vi "Basic ITC-Init2.vi"(0 "Connection Details":T6={"VISA resource name"="", "Comms Layer"=enum."Ethernet TCP/IP", "IP Address"="", "Serial Configuration"={"Baud Rate"=115200, "Parity"=0, "Data Bits"=8, "Stop Bits"=10, "Flow Control"=0}, "ISOBUS address"=-1} {"Serial Configuration"."Flow Control" items=["None", "XON/XOFF", "RTS/CTS", "XON/XOFF & RTS/CTS", "DTR/DSR", "XON/XOFF & DTR/DSR"]; "Serial Configuration"."Stop Bits" items=["1.0"=10, "2.0"=20]; "Serial Configuration"."Data Bits" items=["7"=7, "8"=8]; "Serial Configuration"."Parity" items=["None", "Odd", "Even"]; "Serial Configuration"."Baud Rate" items=["300"=300, "600"=600, "1200"=1200, "2400"=2400, "4800"=4800, "9600"=9600, "14400"=14400, "19200"=19200, "38400"=38400, "57600"=57600, "115200"=115200]}, 7 "ID Query (True)":bool, 9 "Clear Previous Connections (False)":bool, 11 "error in (no error)":errorcluster) -> (1 "Temp Dev Settings Array":T10[](array[typedef]), 2 "Heater Device Settings Array":T19[](array[typedef]), 3 "Device Details":T2, 4 "Merc Ref Out":T8, 6 "Device_ref_Array":T8[](array[typedef]), 8 "Ch_Info":T7, 10 "Pressure Device Settings Array":T31[](array[typedef]), 12 "ISOBUS address":T5=-1, 13 "Aux Device Settings Array":T21[](array[typedef]) {"Signals"."% Open" min=0.0 max=100.0 step=0.1 format="%.4f"; "Signals"."Position" max=20.0 step=1.0 format="%.4f"; "Speed" max=7 step=1; "Gear" max=7 step=1; "Temp V Err" min=0.0 max=20.0 step=0.1; "Temp Err" min=0.0 max=20.0 step=0.1; "Scaling Factor" min=0.0 max=99.0 step=0.1; "Min Flow" min=0.0 max=20.0 step=0.1}, 14 "Level Device Settings Array":T23[](array[typedef]), 15 "error out":errorcluster)   [LabVIEW 2013]
uses:
  <instrlib>/Mercury iXX/Public/Controls/Comms Transport Layer.ctl
  <instrlib>/Mercury iXX/Public/Controls/Serial Settings.ctl
  <instrlib>/Mercury iXX/Public/Controls/ISOBus Address.ctl
  <instrlib>/Mercury iXX/Public/Controls/Mercury Reference.ctl
  <instrlib>/Mercury iXX/Private/Controls/Query Dynamic Reference.ctl
  <instrlib>/Mercury iXX/Public/Libraries/Temperature/Controls/Temperature Device (Read).ctl
  <instrlib>/Mercury iXX/Public/Controls/Manufacturing Data.ctl
  <instrlib>/Mercury iXX/Public/Libraries/Temperature/Controls/Temperature Sensor Type.ctl
  <instrlib>/Mercury iXX/Public/Libraries/Temperature/Controls/Excitation Cluster.ctl
  <instrlib>/Mercury iXX/Public/Libraries/Temperature/Controls/Excitation Type.ctl
  <instrlib>/Mercury iXX/Public/Libraries/Temperature/Controls/Calibration Cluster.ctl
  <instrlib>/Mercury iXX/Public/Libraries/Temperature/Controls/Calibration Interpolation.ctl
  <instrlib>/Mercury iXX/Public/Libraries/Temperature/Controls/Loop Cluster.ctl
  <instrlib>/Mercury iXX/Public/Libraries/Temperature/Controls/Temperature Signals Cluster.ctl
  <instrlib>/Mercury iXX/Public/Libraries/Heater/Controls/Heater Device (Read).ctl
  <instrlib>/Mercury iXX/Public/Libraries/Heater/Controls/Heater Signals Cluster.ctl
  <instrlib>/Mercury iXX/Public/Libraries/Auxiliary/Controls/AUX Device (Read).ctl
  <instrlib>/Mercury iXX/Public/Libraries/Auxiliary/Controls/AUX Signals (Read).ctl
  <instrlib>/Mercury iXX/Public/Libraries/Level Meter/Controls/Level Meter (Read).ctl
  <instrlib>/Mercury iXX/Public/Libraries/Level Meter/Controls/Nitrogen Configuration.ctl
  <instrlib>/Mercury iXX/Public/Libraries/Level Meter/Controls/Frequency Configuration.ctl
  <instrlib>/Mercury iXX/Public/Libraries/Level Meter/Controls/Signals.ctl
  <instrlib>/Mercury iXX/Public/Libraries/Level Meter/Controls/Helium Configuration.ctl
  <instrlib>/Mercury iXX/Public/Libraries/Level Meter/Controls/Resistance Configuration.ctl
  <instrlib>/Mercury iXX/Public/Libraries/Level Meter/Controls/Pre-Pulse.ctl
  <instrlib>/Mercury iXX/Public/Libraries/Level Meter/Controls/Pulse.ctl
  <instrlib>/Mercury iXX/Public/Libraries/Pressure/Controls/Pressure Device (Read).ctl
  <instrlib>/Mercury iXX/Public/Libraries/Pressure/Controls/Pressure Sensor Type.ctl
  <instrlib>/Mercury iXX/Public/Libraries/Pressure/Controls/Calibration Cluster.ctl
  <instrlib>/Mercury iXX/Public/Libraries/Pressure/Controls/Calibration Interpolation.ctl
  <instrlib>/Mercury iXX/Public/Libraries/Pressure/Controls/Loop Cluster.ctl
  <instrlib>/Mercury iXX/Public/Libraries/Pressure/Controls/Pressure Signals Cluster.ctl
  <instrlib>/Mercury iXX/Public/Libraries/System/Open/Open System.vi
  <instrlib>/Mercury iXX/Public/Libraries/System/Read/Catalogue (Read).vi
  <instrlib>/Mercury iXX/Public/Libraries/System/Read/DateTime (Read).vi
  <instrlib>/Mercury iXX/Mercury iXX.lvlib
  <instrlib>/Mercury iXX/Public/Libraries/System.lvlib
  <instrlib>/Mercury iXX/Public/Libraries/Temperature.lvlib
  <instrlib>/Mercury iXX/Public/Libraries/Heater.lvlib
  <instrlib>/Mercury iXX/Public/Libraries/Auxiliary.lvlib
  <instrlib>/Mercury iXX/Public/Libraries/Level Meter.lvlib
  <instrlib>/Mercury iXX/Public/Libraries/Pressure.lvlib
panel:
  in  "Tab Control":T1(tab)
  out "Sys_time_stamp":timestamp
  # "MB0\nMB1\nDB1\nDB2\nDB3\nDB4\nDB5\nDB6\nDB7\nDB8"
  # "Type 0 = Temp\nType 1 = Heater\nType 2 = Aux/gas\nType 3 = Level\nType 4 = Press\nType 5 = Empty"
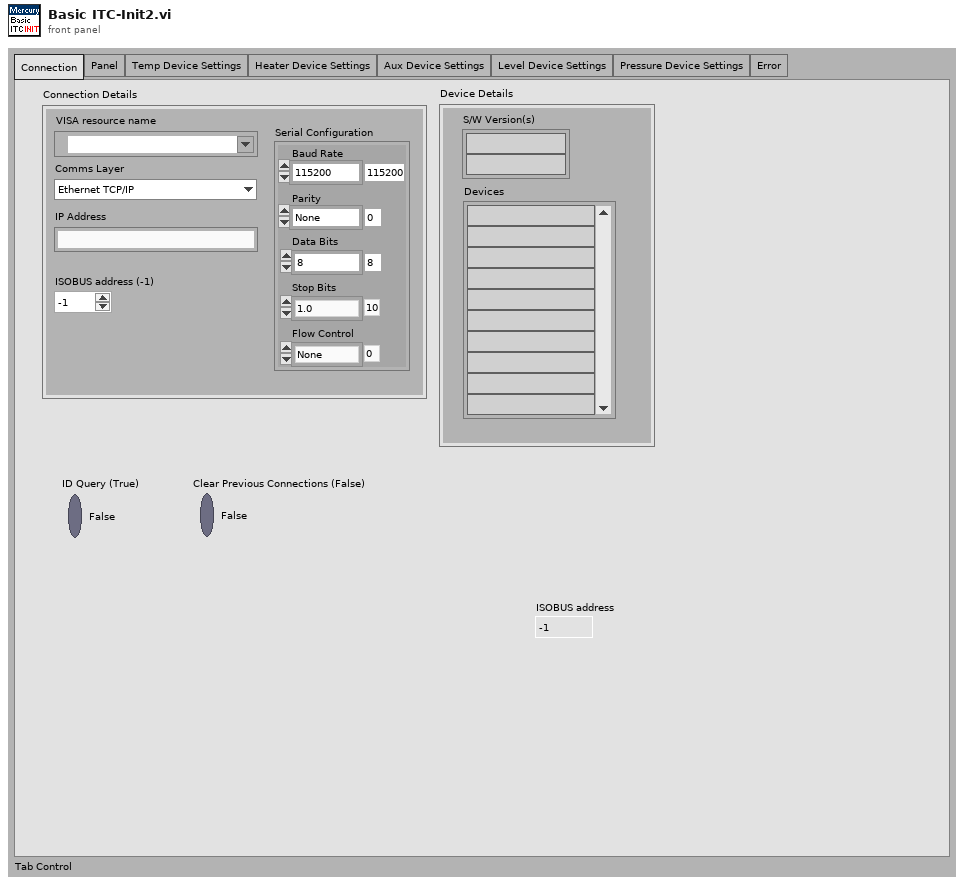
[diagram p1: front panel]
types:
  T1 = enum32{"Connection", "Panel", "Temp Device Settings", "Heater Device Settings", "Aux Device Settings", "Level Device Settings", "Pressure Device Settings", "Error"}
  T2 = cluster{"Devices":string[], "S/W Version(s)":string[]}
  T3 = typedef "Mercury iXX.lvlib/Comms Transport Layer.ctl" = enum16{"Ethernet TCP/IP", "USB", "ISOBus - RS-232", "GPIB"}
  T4 = typedef "Mercury iXX.lvlib/Serial Settings.ctl" = cluster{"Baud Rate":u32, "Parity":u16, "Data Bits":u16, "Stop Bits":u16, "Flow Control":u16}
  T5 = typedef "Mercury iXX.lvlib/ISOBus Address.ctl" = i32
  T6 = cluster{"VISA resource name":refnum<visa-resource-name>, "Comms Layer":T3, "IP Address":string, "Serial Configuration":T4, "ISOBUS address":T5}
  T7 = cluster{"Device_Present?":bool[], "Ch_type_index":i32[]}
  T8 = typedef "Mercury iXX.lvlib/Mercury Reference.ctl" = cluster{"Comms":refnum<visa-resource-name>, "Device ID":string[], "Comms Layer":T3, "Command":string, "Query reference":T9}
  T9 = typedef "Mercury iXX.lvlib/Query Dynamic Reference.ctl" = refnum<vi>
  T10 = typedef "Mercury iXX.lvlib/Temperature.lvlib/Temperature Device (Read).ctl" = cluster{"Manufacturing":T11, "Temperature Sensor Type":T12, "Excitation":T13, "Calibration":T15, "Control Loop":T17, "Temperature Signals":T18, "Nickname":string, "Status":string}
  T11 = typedef "Mercury iXX.lvlib/Manufacturing Data.ctl" = cluster{"Hardware Version":string, "Firmware Version":string, "Serial Number":string}
  T12 = typedef "Mercury iXX.lvlib/Temperature.lvlib/Temperature Sensor Type.ctl" = string
  T13 = typedef "Mercury iXX.lvlib/Temperature.lvlib/Excitation Cluster.ctl" = cluster{"Excitation Type":T14, "Magnitude":string}
  T14 = typedef "Mercury iXX.lvlib/Temperature.lvlib/Excitation Type.ctl" = string
  T15 = typedef "Mercury iXX.lvlib/Temperature.lvlib/Calibration Cluster.ctl" = cluster{"Filename":string, "Interpolation":T16, "Scaling Factor":string, "Offset Factor":string, "Hot Limit":string, "Cold Limit":string, "Last Calibration":string, "Reference":string}
  T16 = typedef "Mercury iXX.lvlib/Temperature.lvlib/Calibration Interpolation.ctl" = string
  T17 = typedef "Mercury iXX.lvlib/Temperature.lvlib/Loop Cluster.ctl" = cluster{"Heater":string, "Auxiliary":string, "Heater Auto":string, "Percentage Heat":string, "Temperature Set Point":string, "PID Auto (from file)":string, "P Value":string, "I Value":string, "D Value":string, "Auto PID Table Filename":string, "Flow Auto":string, "Target Heater Table":string, "Sweep mode":string, "Sweep Table Filename":string, "Percentage Flow":string}
  T18 = typedef "Mercury iXX.lvlib/Temperature.lvlib/Temperature Signals Cluster.ctl" = cluster{"Voltage":string, "Current":string, "Power":string, "Resistance":string, "Temperature":string, "Sensitivity":string, "Reference":string}
  T19 = typedef "Mercury iXX.lvlib/Heater.lvlib/Heater Device (Read).ctl" = cluster{"Manufacturing":T11, "Nickname":string, "Voltage Limit":string, "Nominal Resistance":string, "Maximum Power":string, "Heater Signals":T20, "Status":string}
  T20 = typedef "Mercury iXX.lvlib/Heater.lvlib/Heater Signals Cluster.ctl" = cluster{"Voltage":string, "Current":string, "Power":string}
  T21 = typedef "Mercury iXX.lvlib/Auxiliary.lvlib/AUX Device (Read).ctl" = cluster{"Manufacturing":T11, "Min Flow":dbl, "Scaling Factor":dbl, "Temp Err":dbl, "Temp V Err":dbl, "Gear":u32, "Speed":u32, "Signals":T22, "Nickname":string, "Status":string}
  T22 = typedef "Mercury iXX.lvlib/Auxiliary.lvlib/AUX Signals (Read).ctl" = cluster{"Position":dbl, "% Open":dbl, "I0":string, "I1":string, "I2":string, "I3":string, "O0":string, "O1":string, "O2":string, "O3":string}
  T23 = typedef "Mercury iXX.lvlib/Level Meter.lvlib/Level Meter (Read).ctl" = cluster{"Manufacturing":T11, "Nitrogen Configuration":T24, "Signals":T26, "Nickname":string, "Status":string, "Helium Configuration":T27}
  T24 = typedef "Mercury iXX.lvlib/Level Meter.lvlib/Nitrogen Configuration.ctl" = cluster{"Frequency Configuration":T25, "Pulse Period":dbl}
  T25 = typedef "Mercury iXX.lvlib/Level Meter.lvlib/Frequency Configuration.ctl" = cluster{"Freq 0%":dbl, "Freq 100%":dbl}
  T26 = typedef "Mercury iXX.lvlib/Level Meter.lvlib/Signals.ctl" = cluster{"Helium Signals":cluster{"Resistance":dbl, "Level":dbl}, "Nitrogen Signals":cluster{"Count":dbl, "Freq":dbl, "Level":dbl}}
  T27 = typedef "Mercury iXX.lvlib/Level Meter.lvlib/Helium Configuration.ctl" = cluster{"Resistance Configuration":T28, "Pre-Pulse":T29, "Pulse":T30}
  T28 = typedef "Mercury iXX.lvlib/Level Meter.lvlib/Resistance Configuration.ctl" = cluster{"Res 0%":dbl, "Res 100%":dbl}
  T29 = typedef "Mercury iXX.lvlib/Level Meter.lvlib/Pre-Pulse.ctl" = cluster{"Magnitude":dbl, "Duration":dbl}
  T30 = typedef "Mercury iXX.lvlib/Level Meter.lvlib/Pulse.ctl" = cluster{"Magnitude":dbl, "Duration":dbl, "Delay":dbl}
  T31 = typedef "Mercury iXX.lvlib/Pressure.lvlib/Pressure Device (Read).ctl" = cluster{"Manufacturing":T11, "Temperature Sensor Type":T32, "Calibration":T33, "Control Loop":T35, "Pressure Signals":T36, "Nickname":string, "Status":string}
  T32 = typedef "Mercury iXX.lvlib/Pressure.lvlib/Pressure Sensor Type.ctl" = string
  T33 = typedef "Mercury iXX.lvlib/Pressure.lvlib/Calibration Cluster.ctl" = cluster{"Filename":string, "Interpolation":T34, "Scaling Factor":string, "Offset Factor":string, "High Limit":string, "Low Limit":string, "Last Calibration":string}
  T34 = typedef "Mercury iXX.lvlib/Pressure.lvlib/Calibration Interpolation.ctl" = string
  T35 = typedef "Mercury iXX.lvlib/Pressure.lvlib/Loop Cluster.ctl" = cluster{"Heater":string, "Auxiliary":string, "Heater Auto":string, "Percentage Heat":string, "Pressure Set Point":string, "PID Auto (from file)":string, "P Value":string, "I Value":string, "D Value":string, "Auto PID Table Filename":string, "Flow Auto":string, "Target Heater Table":string, "Sweep mode":string, "Sweep Table Filename":string, "Percentage Flow":string}
  T36 = typedef "Mercury iXX.lvlib/Pressure.lvlib/Pressure Signals Cluster.ctl" = cluster{"Voltage":string, "Current":string, "Power":string, "Pressure":string}
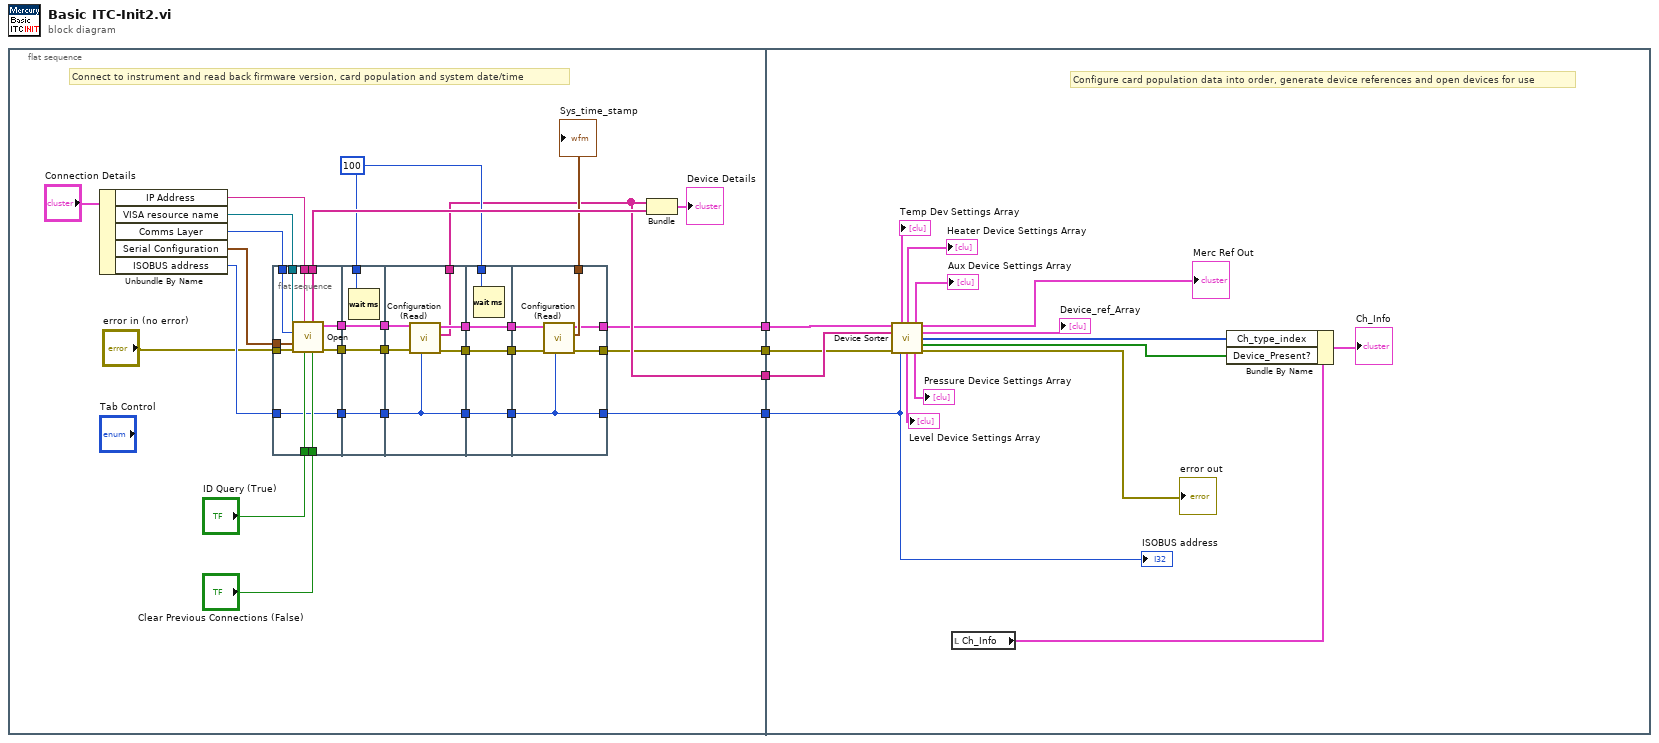
[diagram p0: block diagram]
diagram:
  n1 = flat-sequence {
    tunnel: [w8] -> w4
    tunnel: [w7] -> w3
    tunnel: [w6] -> w2
    tunnel: [w5] -> w1
    tunnel: w4 -> [w80]
    tunnel: w3 -> [w78]
    tunnel: w2 -> [w79]
    tunnel: w1 -> [w69]
    frame #0 {
      w11 = i16 100 ("Interval between messages (ms)")
      # "Connect to instrument and read back firmware version, card population and system date/time"
      n2 = Unbundle By Name("Connection Details") -> ("IP Address"=w17:string, "VISA resource name"=w16:refnum<visa-resource-name>, "Comms Layer"=w15:T3, "Serial Configuration"=w18:T4, "ISOBUS address"=w12:T5)
      n3 = flat-sequence {
        tunnel: "error in (no error)" -> [w44]
        tunnel: "ID Query (True)" -> [w43]
        tunnel: "Clear Previous Connections (False)" -> [w42]
        tunnel: w18 -> [w39]
        tunnel: w17 -> [w38]
        tunnel: w16 -> [w37]
        tunnel: w15 -> [w36]
        tunnel: [w35] -> w13
        tunnel: [w41] -> w33
        tunnel: [w40] -> w32
        tunnel: w12 -> [w34]
        tunnel: [w34] -> w31
        tunnel: w33 -> [w48]
        tunnel: w32 -> [w47]
        tunnel: [w48] -> w30
        tunnel: [w47] -> w29
        tunnel: w31 -> [w46]
        tunnel: [w46] -> w28
        tunnel: w11 -> [w45]
        tunnel: w30 -> [w53]
        tunnel: w29 -> [w52]
        tunnel: w28 -> [w54]
        tunnel: [w54] -> w27
        tunnel: [w51] -> w26
        tunnel: [w50] -> w25
        tunnel: [w49] -> w8
        tunnel: w27 -> [w58]
        tunnel: w26 -> [w57]
        tunnel: w25 -> [w56]
        tunnel: w11 -> [w55]
        tunnel: [w58] -> w24
        tunnel: [w57] -> w23
        tunnel: [w56] -> w22
        tunnel: w24 -> [w62]
        tunnel: w23 -> [w63]
        tunnel: w22 -> [w64]
        tunnel: [w61] -> w10
        tunnel: [w62] -> w5
        tunnel: [w60] -> w7
        tunnel: [w59] -> w6
        frame #0 {
          n4 = call-poly <instrlib>:"Open.vi"("Clear Previous Connections (False)"=w42, "ID Query (True)"=w43, "IP Address"=w38, "error in (no error)"=w44, "Serial Configuration"=w39, "Comms Layer"=w36, "VISA resource name"=w37) -> ("error out"=w40:errorcluster, "Mercury Reference Out"=w41:T8, "S/W Version(s)"=w35:string[])  [unwired: 2 out]
        }
        frame #1 {
          n5 = Wait (ms)(milliseconds to wait=w45) -> ()  [unwired: 1 out]
        }
        frame #2 {
          n6 = call-poly <instrlib>:"Configuration (Read).vi"("ISOBUS address"=w54, "error in"=w52, "Mercury Reference In"=w53) -> ("error out"=w51:errorcluster, "Devices"=w49:string[], "Mercury Reference Out"=w50:T8)  [unwired: 6 out]
        }
        frame #3 {
          n7 = Wait (ms)(milliseconds to wait=w55) -> ()  [unwired: 1 out]
        }
        frame #4 {
          n8 = call-poly <instrlib>:"Configuration (Read).vi"("ISOBUS address"=w62, "error in"=w63, "Mercury Reference In"=w64) -> ("error out"=w59:errorcluster, "time stamp"=w61:timestamp, "Mercury Reference Out"=w60:T8)  [unwired: 6 out]
        }
      }
      n9 = Bundle("Devices"=w8, "S/W Version(s)"=w13) -> (→"Device Details":T2)  [unwired: 1 out]
      "Sys_time_stamp" <- w10
    }
    frame #1 {
      # "Configure card population data into order, generate device references and open devices for use"
      n10 = call <instrlib>:"Device Sorter.vi"("Mercury Ref"=w78, "Devices"=w80, "error in"=w79, "ISOBUS address"=w69) -> ("Temp Dev Settings Array"=→"Temp Dev Settings Array":T10[], "Heater Device Settings Array"=→"Heater Device Settings Array":T19[], "Aux Device Settings Array"=→"Aux Device Settings Array":T21[], "Mercury Ref Out"=→"Merc Ref Out":T8, "Device_ref_Array"=→"Device_ref_Array":T8[], "Ch_type_index"=w67:i32[], "Device_Present?"=w66:bool[], "Level Device Settings Array"=→"Level Device Settings Array":T23[], "Pressure Device Settings Array"=→"Pressure Device Settings Array":T31[], "error out"=→"error out":errorcluster)  [unwired: 2 in]
      n11 = local read "Ch_Info"() -> (w68:T7)
      n12 = Bundle By Name(cluster=w68, "Ch_type_index"=w67, "Device_Present?"=w66) -> (→"Ch_Info":T7)
      "ISOBUS address" <- w69
    }
  }
